vi "MRC Ds Comms Get Joystick Descriptors.vi"(8 "error in (no error)":errorcluster) -> (0 "error out":errorcluster, 3 "joystickDescriptors out":T2)   [LabVIEW 2026, in "MrcLib.lvlib"]
doc: "MRC_Status MRC_CALLCONV MRC_DsComms_GetJoystickDescriptors(struct MRC_JoystickDescriptors* joystickDescriptors);"
uses:
  MrcLib.lvlib
  <vilib>/MRC/Types/MRC Str255.ctl
  MrcLib.so
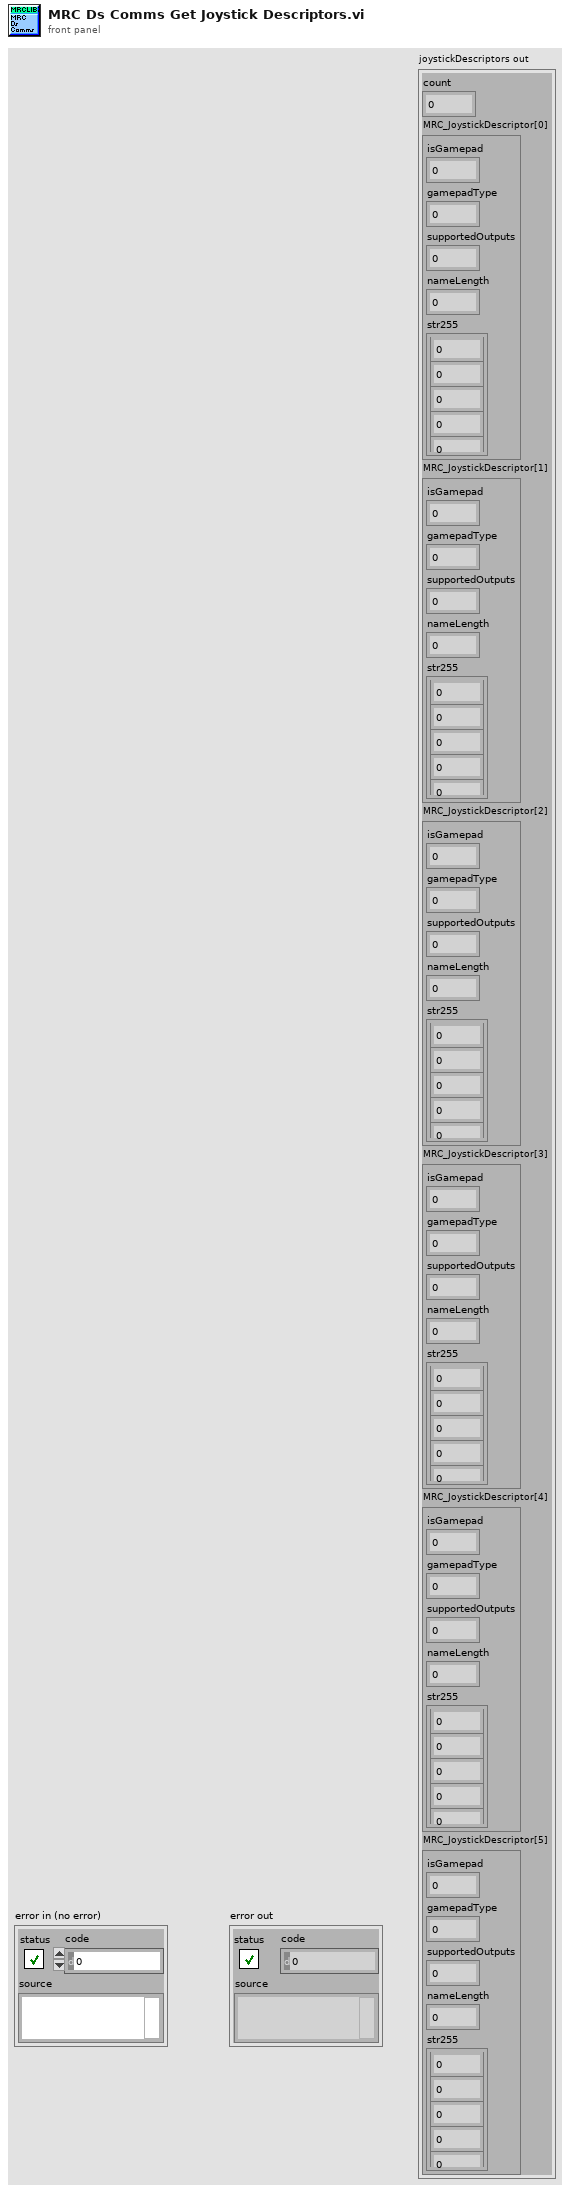
[diagram p1: front panel]
types:
  T1 = typedef "MRC Str255.ctl" = cluster{"[1]":u8, "[2]":u8, "[3]":u8, "[4]":u8, "[5]":u8, "[6]":u8, "[7]":u8, "[8]":u8, "[9]":u8, "[10]":u8, "[11]":u8, "[12]":u8, "[13]":u8, "[14]":u8, "[15]":u8, "[16]":u8, "[17]":u8, "[18]":u8, "[19]":u8, "[20]":u8, "[21]":u8, "[22]":u8, "[23]":u8, "[24]":u8, "[25]":u8, "[26]":u8, "[27]":u8, "[28]":u8, "[29]":u8, "[30]":u8, "[31]":u8, "[32]":u8, "[33]":u8, "[34]":u8, "[35]":u8, "[36]":u8, "[37]":u8, "[38]":u8, "[39]":u8, "[40]":u8, "[41]":u8, "[42]":u8, "[43]":u8, "[44]":u8, "[45]":u8, "[46]":u8, "[47]":u8, "[48]":u8, "[49]":u8, "[50]":u8, "[51]":u8, "[52]":u8, "[53]":u8, "[54]":u8, "[55]":u8, "[56]":u8, "[57]":u8, "[58]":u8, "[59]":u8, "[60]":u8, "[61]":u8, "[62]":u8, "[63]":u8}
  T2 = cluster{"count":u8, "MRC_JoystickDescriptor[0]":cluster{"isGamepad":u8, "gamepadType":u8, "supportedOutputs":u8, "nameLength":u8, "str255":T1}, "MRC_JoystickDescriptor[1]":cluster{"isGamepad":u8, "gamepadType":u8, "supportedOutputs":u8, "nameLength":u8, "str255":T1}, "MRC_JoystickDescriptor[2]":cluster{"isGamepad":u8, "gamepadType":u8, "supportedOutputs":u8, "nameLength":u8, "str255":T1}, "MRC_JoystickDescriptor[3]":cluster{"isGamepad":u8, "gamepadType":u8, "supportedOutputs":u8, "nameLength":u8, "str255":T1}, "MRC_JoystickDescriptor[4]":cluster{"isGamepad":u8, "gamepadType":u8, "supportedOutputs":u8, "nameLength":u8, "str255":T1}, "MRC_JoystickDescriptor[5]":cluster{"isGamepad":u8, "gamepadType":u8, "supportedOutputs":u8, "nameLength":u8, "str255":T1}}
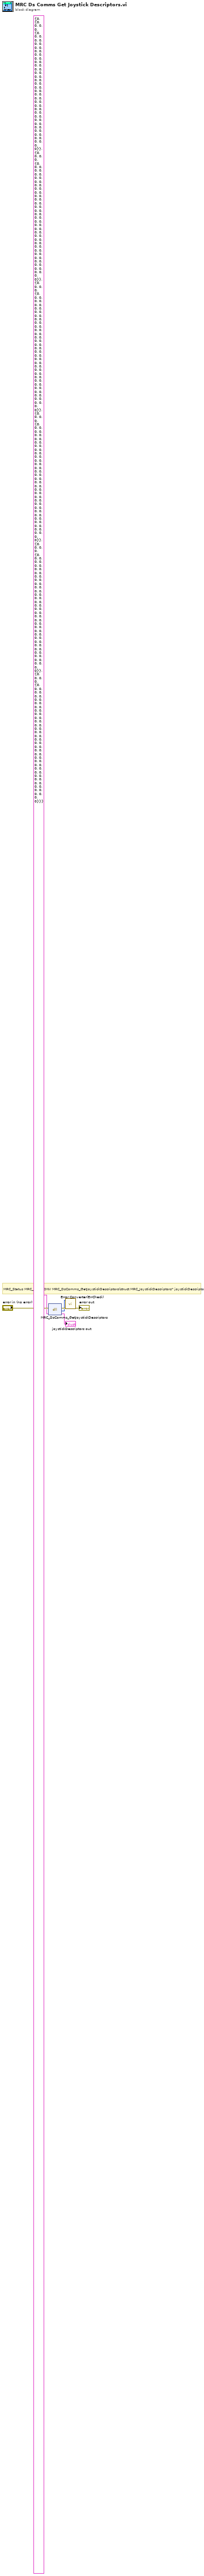
[diagram p0: block diagram]
diagram:
  # "MRC_Status MRC_CALLCONV MRC_DsComms_GetJoystickDescriptors(struct MRC_JoystickDescriptors* joystickDescriptors);"
  n1 = dll-call lib="MrcLib.*" fn="MRC_DsComms_GetJoystickDescriptors"(error in="error in (no error)", T2 {"count"=0, "MRC_JoystickDescriptor[0]"={"isGamepad"=0, "gamepadType"=0, "supportedOutputs"=0, "nameLength"=0, "str255"={"[1]"=0, "[2]"=0, "[3]"=0, "[4]"=0, "[5]"=0, "[6]"=0, "[7]"=0, "[8]"=0, "[9]"=0, "[10]"=0, "[11]"=0, "[12]"=0, "[13]"=0, "[14]"=0, "[15]"=0, "[16]"=0, "[17]"=0, "[18]"=0, "[19]"=0, "[20]"=0, "[21]"=0, "[22]"=0, "[23]"=0, "[24]"=0, "[25]"=0, "[26]"=0, "[27]"=0, "[28]"=0, "[29]"=0, "[30]"=0, "[31]"=0, "[32]"=0, "[33]"=0, "[34]"=0, "[35]"=0, "[36]"=0, "[37]"=0, "[38]"=0, "[39]"=0, "[40]"=0, "[41]"=0, "[42]"=0, "[43]"=0, "[44]"=0, "[45]"=0, "[46]"=0, "[47]"=0, "[48]"=0, "[49]"=0, "[50]"=0, "[51]"=0, "[52]"=0, "[53]"=0, "[54]"=0, "[55]"=0, "[56]"=0, "[57]"=0, "[58]"=0, "[59]"=0, "[60]"=0, "[61]"=0, "[62]"=0, "[63]"=0}}, "MRC_JoystickDescriptor[1]"={"isGamepad"=0, "gamepadType"=0, "supportedOutputs"=0, "nameLength"=0, "str255"={"[1]"=0, "[2]"=0, "[3]"=0, "[4]"=0, "[5]"=0, "[6]"=0, "[7]"=0, "[8]"=0, "[9]"=0, "[10]"=0, "[11]"=0, "[12]"=0, "[13]"=0, "[14]"=0, "[15]"=0, "[16]"=0, "[17]"=0, "[18]"=0, "[19]"=0, "[20]"=0, "[21]"=0, "[22]"=0, "[23]"=0, "[24]"=0, "[25]"=0, "[26]"=0, "[27]"=0, "[28]"=0, "[29]"=0, "[30]"=0, "[31]"=0, "[32]"=0, "[33]"=0, "[34]"=0, "[35]"=0, "[36]"=0, "[37]"=0, "[38]"=0, "[39]"=0, "[40]"=0, "[41]"=0, "[42]"=0, "[43]"=0, "[44]"=0, "[45]"=0, "[46]"=0, "[47]"=0, "[48]"=0, "[49]"=0, "[50]"=0, "[51]"=0, "[52]"=0, "[53]"=0, "[54]"=0, "[55]"=0, "[56]"=0, "[57]"=0, "[58]"=0, "[59]"=0, "[60]"=0, "[61]"=0, "[62]"=0, "[63]"=0}}, "MRC_JoystickDescriptor[2]"={"isGamepad"=0, "gamepadType"=0, "supportedOutputs"=0, "nameLength"=0, "str255"={"[1]"=0, "[2]"=0, "[3]"=0, "[4]"=0, "[5]"=0, "[6]"=0, "[7]"=0, "[8]"=0, "[9]"=0, "[10]"=0, "[11]"=0, "[12]"=0, "[13]"=0, "[14]"=0, "[15]"=0, "[16]"=0, "[17]"=0, "[18]"=0, "[19]"=0, "[20]"=0, "[21]"=0, "[22]"=0, "[23]"=0, "[24]"=0, "[25]"=0, "[26]"=0, "[27]"=0, "[28]"=0, "[29]"=0, "[30]"=0, "[31]"=0, "[32]"=0, "[33]"=0, "[34]"=0, "[35]"=0, "[36]"=0, "[37]"=0, "[38]"=0, "[39]"=0, "[40]"=0, "[41]"=0, "[42]"=0, "[43]"=0, "[44]"=0, "[45]"=0, "[46]"=0, "[47]"=0, "[48]"=0, "[49]"=0, "[50]"=0, "[51]"=0, "[52]"=0, "[53]"=0, "[54]"=0, "[55]"=0, "[56]"=0, "[57]"=0, "[58]"=0, "[59]"=0, "[60]"=0, "[61]"=0, "[62]"=0, "[63]"=0}}, "MRC_JoystickDescriptor[3]"={"isGamepad"=0, "gamepadType"=0, "supportedOutputs"=0, "nameLength"=0, "str255"={"[1]"=0, "[2]"=0, "[3]"=0, "[4]"=0, "[5]"=0, "[6]"=0, "[7]"=0, "[8]"=0, "[9]"=0, "[10]"=0, "[11]"=0, "[12]"=0, "[13]"=0, "[14]"=0, "[15]"=0, "[16]"=0, "[17]"=0, "[18]"=0, "[19]"=0, "[20]"=0, "[21]"=0, "[22]"=0, "[23]"=0, "[24]"=0, "[25]"=0, "[26]"=0, "[27]"=0, "[28]"=0, "[29]"=0, "[30]"=0, "[31]"=0, "[32]"=0, "[33]"=0, "[34]"=0, "[35]"=0, "[36]"=0, "[37]"=0, "[38]"=0, "[39]"=0, "[40]"=0, "[41]"=0, "[42]"=0, "[43]"=0, "[44]"=0, "[45]"=0, "[46]"=0, "[47]"=0, "[48]"=0, "[49]"=0, "[50]"=0, "[51]"=0, "[52]"=0, "[53]"=0, "[54]"=0, "[55]"=0, "[56]"=0, "[57]"=0, "[58]"=0, "[59]"=0, "[60]"=0, "[61]"=0, "[62]"=0, "[63]"=0}}, "MRC_JoystickDescriptor[4]"={"isGamepad"=0, "gamepadType"=0, "supportedOutputs"=0, "nameLength"=0, "str255"={"[1]"=0, "[2]"=0, "[3]"=0, "[4]"=0, "[5]"=0, "[6]"=0, "[7]"=0, "[8]"=0, "[9]"=0, "[10]"=0, "[11]"=0, "[12]"=0, "[13]"=0, "[14]"=0, "[15]"=0, "[16]"=0, "[17]"=0, "[18]"=0, "[19]"=0, "[20]"=0, "[21]"=0, "[22]"=0, "[23]"=0, "[24]"=0, "[25]"=0, "[26]"=0, "[27]"=0, "[28]"=0, "[29]"=0, "[30]"=0, "[31]"=0, "[32]"=0, "[33]"=0, "[34]"=0, "[35]"=0, "[36]"=0, "[37]"=0, "[38]"=0, "[39]"=0, "[40]"=0, "[41]"=0, "[42]"=0, "[43]"=0, "[44]"=0, "[45]"=0, "[46]"=0, "[47]"=0, "[48]"=0, "[49]"=0, "[50]"=0, "[51]"=0, "[52]"=0, "[53]"=0, "[54]"=0, "[55]"=0, "[56]"=0, "[57]"=0, "[58]"=0, "[59]"=0, "[60]"=0, "[61]"=0, "[62]"=0, "[63]"=0}}, "MRC_JoystickDescriptor[5]"={"isGamepad"=0, "gamepadType"=0, "supportedOutputs"=0, "nameLength"=0, "str255"={"[1]"=0, "[2]"=0, "[3]"=0, "[4]"=0, "[5]"=0, "[6]"=0, "[7]"=0, "[8]"=0, "[9]"=0, "[10]"=0, "[11]"=0, "[12]"=0, "[13]"=0, "[14]"=0, "[15]"=0, "[16]"=0, "[17]"=0, "[18]"=0, "[19]"=0, "[20]"=0, "[21]"=0, "[22]"=0, "[23]"=0, "[24]"=0, "[25]"=0, "[26]"=0, "[27]"=0, "[28]"=0, "[29]"=0, "[30]"=0, "[31]"=0, "[32]"=0, "[33]"=0, "[34]"=0, "[35]"=0, "[36]"=0, "[37]"=0, "[38]"=0, "[39]"=0, "[40]"=0, "[41]"=0, "[42]"=0, "[43]"=0, "[44]"=0, "[45]"=0, "[46]"=0, "[47]"=0, "[48]"=0, "[49]"=0, "[50]"=0, "[51]"=0, "[52]"=0, "[53]"=0, "[54]"=0, "[55]"=0, "[56]"=0, "[57]"=0, "[58]"=0, "[59]"=0, "[60]"=0, "[61]"=0, "[62]"=0, "[63]"=0}}} ("joystickDescriptors out")) -> (error out=w5:errorcluster, "return type"=w3:i32, →"joystickDescriptors out":T2)  [unwired: 2 in, 1 out]
  n2 = call <vilib>:"Error Converter(ErrCheck).vi"("error in (no error)"=w5, "status"=w3) -> ("error out"=→"error out":errorcluster)  [unwired: 9 in]
